vi "4155C Sample Config SMUs FPP.vi"(8 "error in (no error)":errorcluster, 9 "Drain Standby":bool, 10 "Gate Standby":bool, 11 "VISA resource name in":refnum<visa-resource-name>) -> (0 "error out":errorcluster, 3 "VISA Resource Name out":refnum<visa-resource-name>)   [LabVIEW 2016]
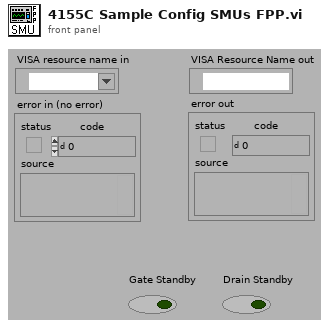
[diagram p1: front panel]
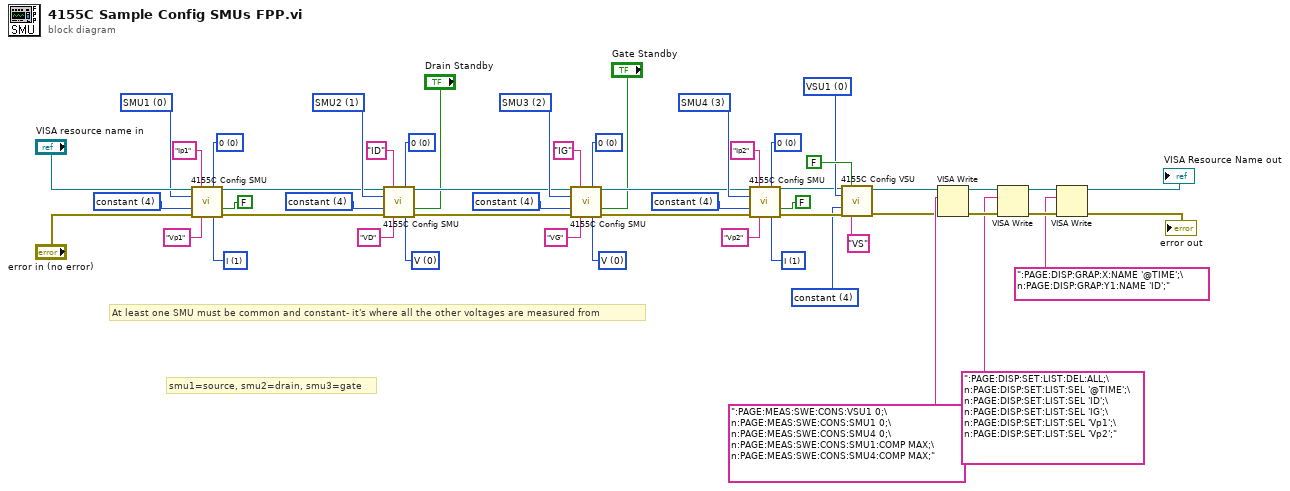
[diagram p0: block diagram]
diagram:
  w15 = u32 0 items=["VSU1  ", "VSU2  "] ("unit to configure")
  w17 = u32 4 items=["disabled  ", "VAR1  ", "VAR2  ", "VAR1'  ", "constant  "] ("function")
  w28 = u32 1 items=["V  ", "I  ", "V pulse  ", "I pulse  ", "  common  "] ("mode")
  w29 = u32 0 items=["0  ", "10K Ohms  ", "100K Ohms  ", "1M Ohms  "] ("series resistance *")
  w31 = u32 4 items=["disabled  ", "VAR1  ", "VAR2  ", "VAR1'  ", "constant  "] ("function")
  w32 = u32 3 items=["SMU1  ", "SMU2  ", "SMU3  ", "SMU4  ", "SMU5  ", "SMU6  "] ("unit to configure")
  w34 = u32 0 items=["V  ", "I  ", "V pulse  ", "I pulse  ", "  common  "] ("mode")
  w35 = u32 0 items=["0  ", "10K Ohms  ", "100K Ohms  ", "1M Ohms  "] ("series resistance *")
  w37 = u32 4 items=["disabled  ", "VAR1  ", "VAR2  ", "VAR1'  ", "constant  "] ("function")
  w38 = u32 2 items=["SMU1  ", "SMU2  ", "SMU3  ", "SMU4  ", "SMU5  ", "SMU6  "] ("unit to configure")
  w40 = u32 0 items=["V  ", "I  ", "V pulse  ", "I pulse  ", "  common  "] ("mode")
  w41 = u32 0 items=["0  ", "10K Ohms  ", "100K Ohms  ", "1M Ohms  "] ("series resistance *")
  w43 = u32 4 items=["disabled  ", "VAR1  ", "VAR2  ", "VAR1'  ", "constant  "] ("function")
  w44 = u32 1 items=["SMU1  ", "SMU2  ", "SMU3  ", "SMU4  ", "SMU5  ", "SMU6  "] ("unit to configure")
  w47 = u32 1 items=["V  ", "I  ", "V pulse  ", "I pulse  ", "  common  "] ("mode")
  w48 = u32 0 items=["0  ", "10K Ohms  ", "100K Ohms  ", "1M Ohms  "] ("series resistance *")
  w50 = u32 4 items=["disabled  ", "VAR1  ", "VAR2  ", "VAR1'  ", "constant  "] ("function")
  w51 = u32 0 items=["SMU1  ", "SMU2  ", "SMU3  ", "SMU4  ", "SMU5  ", "SMU6  "] ("unit to configure")
  # "smu1=source, smu2=drain, smu3=gate"
  # "At least one SMU must be common and constant- it's where all the other voltages are measured from"
  n1 = call "4155C Config SMU.vi"("VISA session"="VISA resource name in", "I name (max 6 chars)"="Ip1", "series resistance *"=w48, "unit to configure"=w51, "function"=w50, "standby"=FALSE, "error in (no error)"="error in (no error)", "V name (max 6 chars)"="Vp1", "mode"=w47) -> ("dup VISA resource name"=w25:refnum<visa-resource-name>, "error out"=w24:errorcluster)  [unwired: 5 in]
  n2 = call "4155C Config SMU.vi"("VISA session"=w25, "I name (max 6 chars)"="ID", "series resistance *"=w41, "unit to configure"=w44, "function"=w43, "standby"="Drain Standby", "error in (no error)"=w24, "V name (max 6 chars)"="VD", "mode"=w40) -> ("dup VISA resource name"=w22:refnum<visa-resource-name>, "error out"=w23:errorcluster)  [unwired: 5 in]
  n3 = call "4155C Config SMU.vi"("VISA session"=w22, "I name (max 6 chars)"="IG", "series resistance *"=w35, "unit to configure"=w38, "function"=w37, "standby"="Gate Standby", "error in (no error)"=w23, "V name (max 6 chars)"="VG", "mode"=w34) -> ("dup VISA resource name"=w21:refnum<visa-resource-name>, "error out"=w20:errorcluster)  [unwired: 5 in]
  n4 = call "4155C Config SMU.vi"("VISA session"=w21, "I name (max 6 chars)"="Ip2", "series resistance *"=w29, "unit to configure"=w32, "function"=w31, "standby"=FALSE, "error in (no error)"=w20, "V name (max 6 chars)"="Vp2", "mode"=w28) -> ("dup VISA resource name"=w14:refnum<visa-resource-name>, "error out"=w19:errorcluster)  [unwired: 5 in]
  n5 = call "4155C Config VSU.vi"("VISA session"=w14, "standby"=FALSE, "unit to configure"=w15, "function"=w17, "error in (no error)"=w19, "V name (max 6 chars)"="VS") -> ("dup VISA resource name"=w11:refnum<visa-resource-name>, "error out"=w12:errorcluster)  [unwired: 8 in]
  n6 = VISA Write(VISA resource name=w11, write buffer=":PAGE:MEAS:SWE:CONS:VSU1 0;\n:PAGE:MEAS:SWE:CONS:SMU1 0;\n:PAGE:MEAS:SWE:CONS:SMU4 0;\n:PAGE:MEAS:SWE:CONS:SMU1:COMP MAX;\n:PAGE:MEAS:SWE:CONS:SMU4:COMP MAX;" ("write buffer (\"\")"), error in (no error)=w12) -> (VISA resource name out=w10:refnum<visa-resource-name>, error out=w5:errorcluster)  [unwired: 1 out]
  n7 = VISA Write(VISA resource name=w10, write buffer=":PAGE:DISP:SET:LIST:DEL:ALL;\n:PAGE:DISP:SET:LIST:SEL '@TIME';\n:PAGE:DISP:SET:LIST:SEL 'ID';\n:PAGE:DISP:SET:LIST:SEL 'IG';\n:PAGE:DISP:SET:LIST:SEL 'Vp1';\n:PAGE:DISP:SET:LIST:SEL 'Vp2';" ("write buffer (\"\")"), error in (no error)=w5) -> (VISA resource name out=w9:refnum<visa-resource-name>, error out=w6:errorcluster)  [unwired: 1 out]
  n8 = VISA Write(VISA resource name=w9, write buffer=":PAGE:DISP:GRAP:X:NAME '@TIME';\n:PAGE:DISP:GRAP:Y1:NAME 'ID';" ("write buffer (\"\")"), error in (no error)=w6) -> (VISA resource name out=→"VISA Resource Name out":refnum<visa-resource-name>, error out=→"error out":errorcluster)  [unwired: 1 out]
